vi "ADO1TEL.vi"() -> ()   [LabVIEW 2018]
panel:
  out "Numeric":dbl
  out "IMC":dbl(knob) scale=0.0..50.0
  out "Morbida - Obsidade G3":bool
  out "Grave - Obsidade G2":bool
  out "Obesidade G1":bool
  out "Sobrepeso":bool
  out "Peso Ideal":bool
  out "Abaixo do peso":bool
  out "Grave - Abaixo do Peso":bool
  out "Extremo - Abaixo do Peso":bool
  out "Altura em m":dbl(knob) scale=0.0..2.5
  out "Peso em KG":dbl(knob) scale=0.0..200.0
  in  "Peso em kg":dbl
  in  "Altura em m":dbl format="%#.6f"
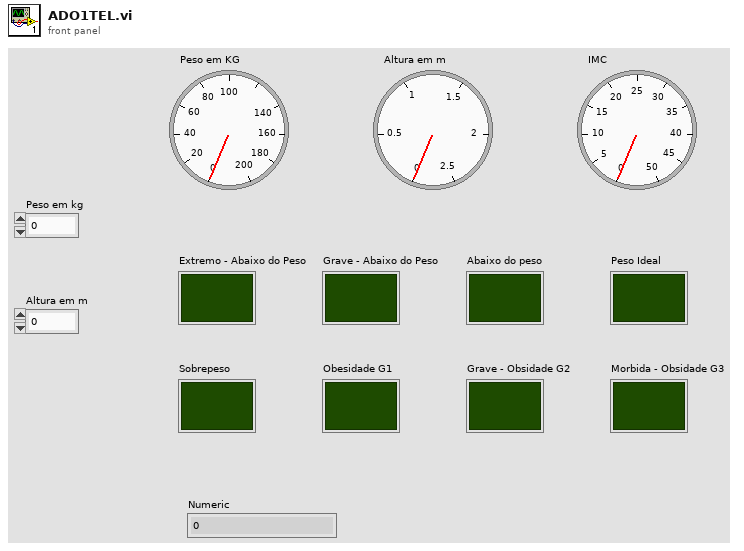
[diagram p1: front panel]
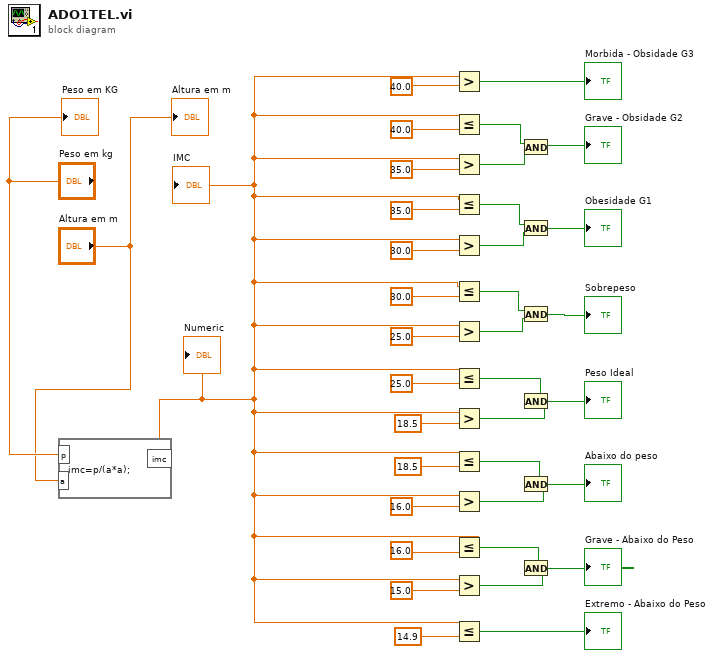
[diagram p0: block diagram]
diagram:
  n1 = formula code="imc=p/(a*a);"("a"="Altura em m", "p"="Peso em kg") -> ("imc"=w2:dbl)
  "IMC" <- w2
  "Numeric" <- w2
  n2 = Greater?(x=w2, y=40.0) -> (0:→"Morbida - Obsidade G3":bool)
  n3 = Less Or Equal?(x=w2, y=40.0) -> (x <= y?=w15:bool)
  n4 = Greater?(x=w2, y=35.0) -> (0:w32:bool)
  n5 = Less Or Equal?(x=w2, y=35.0) -> (x <= y?=w13:bool)
  n6 = Greater?(x=w2, y=30.0) -> (0:w30:bool)
  n7 = Less Or Equal?(x=w2, y=30.0) -> (x <= y?=w12:bool)
  n8 = Greater?(x=w2, y=25.0) -> (0:w28:bool)
  n9 = Less Or Equal?(x=w2, y=25.0) -> (x <= y?=w4:bool)
  n10 = Greater?(x=w2, y=18.5) -> (0:w26:bool)
  n11 = Less Or Equal?(x=w2, y=18.5) -> (x <= y?=w5:bool)
  n12 = Greater?(x=w2, y=16.0) -> (0:w20:bool)
  n13 = Less Or Equal?(x=w2, y=16.0) -> (x <= y?=w8:bool)
  n14 = Greater?(x=w2, y=15.0) -> (0:w24:bool)
  n15 = Less Or Equal?(x=w2, y=14.9) -> (x <= y?=→"Extremo - Abaixo do Peso":bool)
  n16 = And(x=w15, y=w32) -> (x .and. y?=→"Grave - Obsidade G2":bool)
  n17 = And(x=w13, y=w30) -> (x .and. y?=→"Obesidade G1":bool)
  n18 = And(x=w12, y=w28) -> (x .and. y?=→"Sobrepeso":bool)
  n19 = And(x=w4, y=w26) -> (x .and. y?=→"Peso Ideal":bool)
  n20 = And(x=w5, y=w20) -> (x .and. y?=→"Abaixo do peso":bool)
  n21 = And(x=w8, y=w24) -> (x .and. y?=→"Grave - Abaixo do Peso":bool)
  "Peso em KG" <- "Peso em kg"
  "Altura em m" <- "Altura em m"
